vi "soundwave_generator_v06_complete_user.vi"() -> ()   [LabVIEW 2019]
uses:
  global.vi
panel:
  in  "Choice Equal":bool
  in  "Choice 2":bool
  in  "Choice 1":bool
  out "choice 2 LED":bool
  out "choice 1 LED":bool
  in  "Repeat Trial":bool
  out "Trial":i32
  out "Protocol Progression":i32(slide) scale=0.0..90.0
  out "Red Light":bool
  out "Green Light":bool
  out "Sound number":string
  # "Trial #"
  # "Which sound did you prefer?"
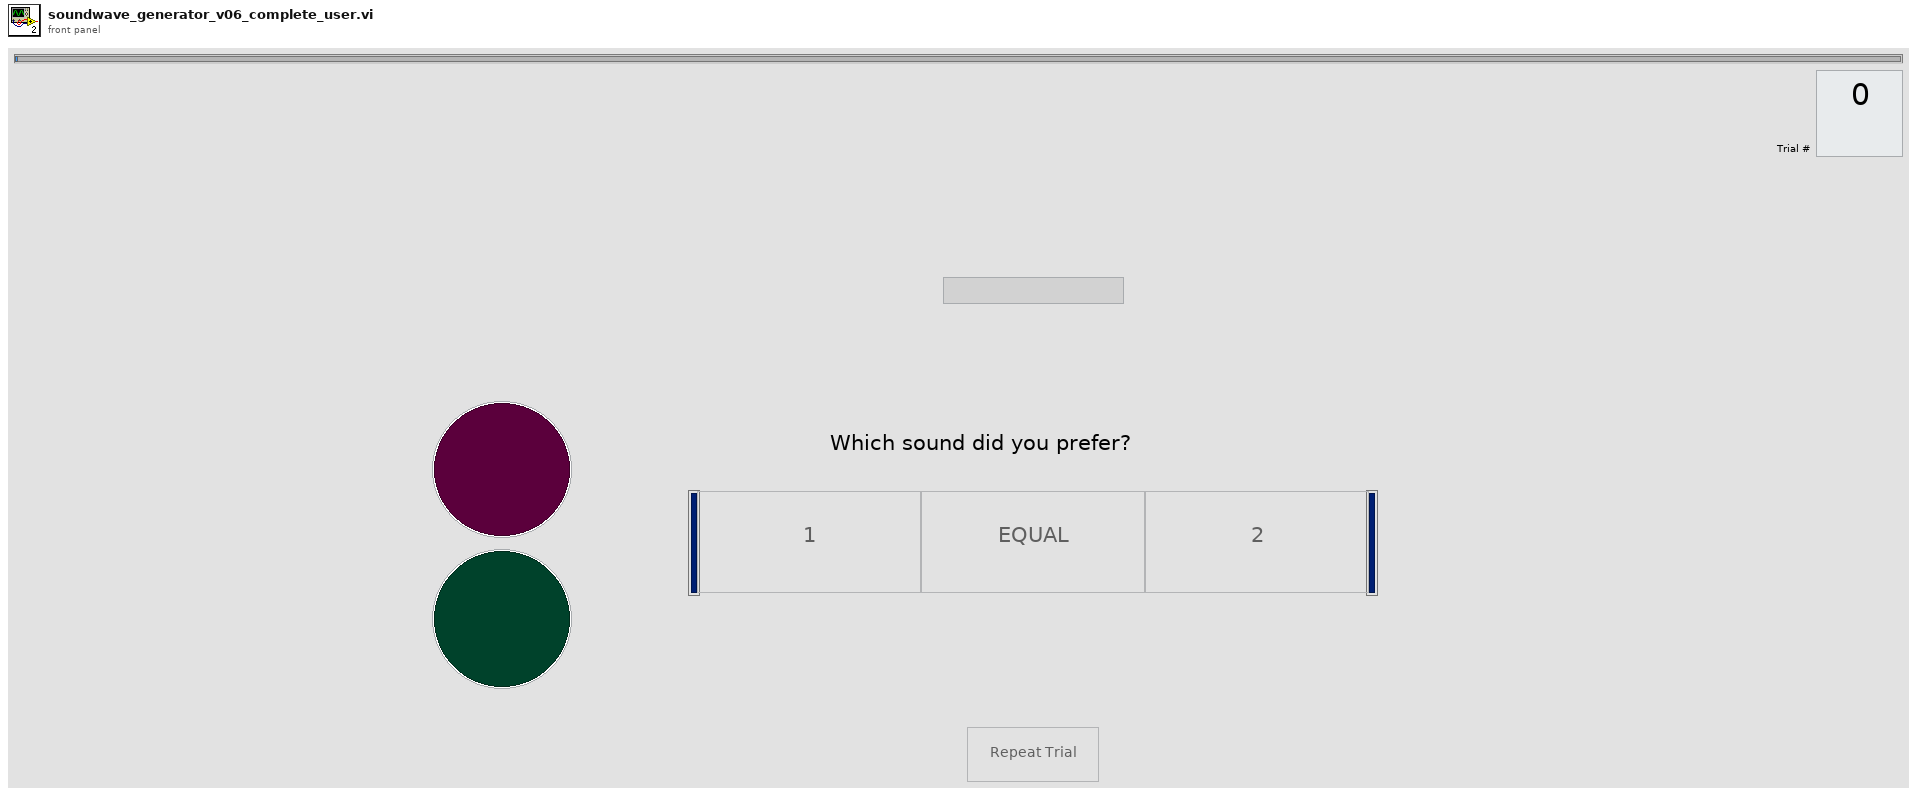
[diagram p1: front panel]
types:
  T1 = enum8{"Enabled", "Disabled", "Disabled and Grayed Out"}
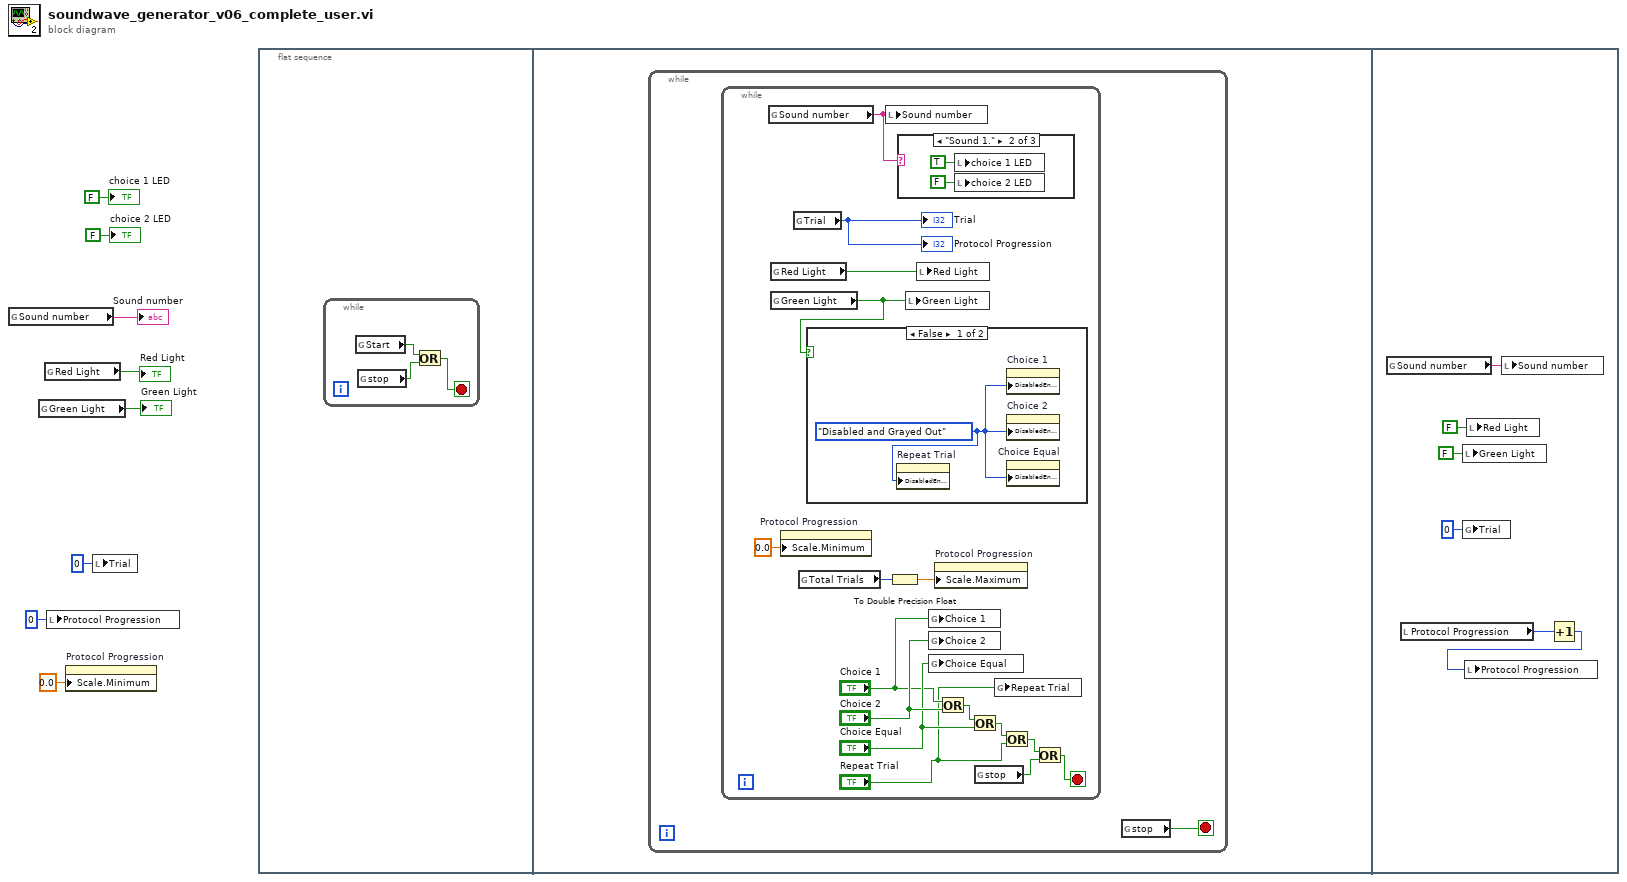
[diagram p0: block diagram]
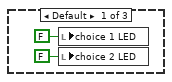
[diagram p2: hidden frame]
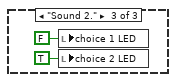
[diagram p3: hidden frame]
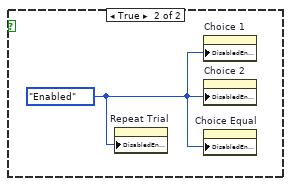
[diagram p4: hidden frame]
diagram:
  n1 = global read "global.vi" "Sound number"() -> (→"Sound number":string)
  n2 = global read "global.vi" "Green Light"() -> (→"Green Light":bool)
  n3 = global read "global.vi" "Red Light"() -> (→"Red Light":bool)
  n4 = local write "Protocol Progression"(0 ("Protocol Progression")) -> ()
  n5 = property on="Protocol Progression" class="Slide (strict)"("Scale.Minimum"=0.0 ("Scale.Range:Minimum")) -> ()  [unwired: 2 in, 2 out]
  n6 = local write "Trial"(0 ("Trial")) -> ()
  n7 = flat-sequence {
    frame #0 {
      n8 = while {
        stop <- w11 stop-if-true
        n9 = global read "global.vi" "Start"() -> (w9:bool)
        n10 = global read "global.vi" "stop"() -> (w10:bool)
        n11 = Or(x=w9, y=w10) -> (x .or. y?=w11:bool)
      }
    }
    frame #1 {
      n12 = while {
        stop <- w12 stop-if-true
        n13 = while {
          stop <- w28 stop-if-true
          n14 = global read "global.vi" "Sound number"() -> (w14:string)
          n15 = global read "global.vi" "Red Light"() -> (w23:bool)
          n16 = global read "global.vi" "Green Light"() -> (w13:bool)
          n17 = property on="Protocol Progression" class="Slide (strict)"("Scale.Minimum"=0.0 ("Scale.Range:Minimum")) -> ()  [unwired: 2 in, 2 out]
          n18 = global read "global.vi" "Trial"() -> (→"Protocol Progression" →"Trial":i32)
          n19 = global read "global.vi" "Total Trials"() -> (w22:i32)
          n20 = case shown="False" w13 {
            frame False {
              w35 = T1."Disabled and Grayed Out" ("Disabled")
              n21 = property on="Repeat Trial" class="Bool"("DisabledEnum"=w35) -> ()  [unwired: 2 in, 2 out]
              n22 = property on="Choice 1" class="Bool"("DisabledEnum"=w35) -> ()  [unwired: 2 in, 2 out]
              n23 = property on="Choice 2" class="Bool"("DisabledEnum"=w35) -> ()  [unwired: 2 in, 2 out]
              n24 = property on="Choice Equal" class="Bool"("DisabledEnum"=w35) -> ()  [unwired: 2 in, 2 out]
            }
            frame True {
              w36 = T1."Enabled" ("Disabled")
              n25 = property on="Repeat Trial" class="Bool"("DisabledEnum"=w36) -> ()  [unwired: 2 in, 2 out]
              n26 = property on="Choice 1" class="Bool"("DisabledEnum"=w36) -> ()  [unwired: 2 in, 2 out]
              n27 = property on="Choice 2" class="Bool"("DisabledEnum"=w36) -> ()  [unwired: 2 in, 2 out]
              n28 = property on="Choice Equal" class="Bool"("DisabledEnum"=w36) -> ()  [unwired: 2 in, 2 out]
            }
          }
          n29 = local write "Sound number"(w14) -> ()
          n30 = To Double Precision Float(number=w22) -> (double precision float=w21:dbl)
          n31 = case shown="\"Sound 1.\"" w14 {
            frame Default {
              n32 = local write "choice 1 LED"(FALSE ("choice 1 LED")) -> ()
              n33 = local write "choice 2 LED"(FALSE ("choice 2 LED")) -> ()
            }
            frame "Sound 1." {
              n34 = local write "choice 1 LED"(TRUE ("choice 1 LED")) -> ()
              n35 = local write "choice 2 LED"(FALSE ("choice 2 LED")) -> ()
            }
            frame "Sound 2." {
              n36 = local write "choice 1 LED"(FALSE ("choice 1 LED")) -> ()
              n37 = local write "choice 2 LED"(TRUE ("choice 2 LED")) -> ()
            }
          }
          n38 = local write "Green Light"(w13) -> ()
          n39 = local write "Red Light"(w23) -> ()
          n40 = global write "global.vi" "Choice 1"("Choice 1") -> ()
          n41 = global write "global.vi" "Choice 2"("Choice 2") -> ()
          n42 = global write "global.vi" "Choice Equal"("Choice Equal") -> ()
          n43 = property on="Protocol Progression" class="Slide (strict)"("Scale.Maximum"=w21) -> ()  [unwired: 2 in, 2 out]
          n44 = Or(x="Choice 1", y="Choice 2") -> (x .or. y?=w27:bool)
          n45 = Or(x=w27, y="Choice Equal") -> (x .or. y?=w18:bool)
          n46 = global read "global.vi" "stop"() -> (w26:bool)
          n47 = global write "global.vi" "Repeat Trial"("Repeat Trial") -> ()
          n48 = Or(x=w18, y="Repeat Trial") -> (x .or. y?=w17:bool)
          n49 = Or(x=w17, y=w26) -> (x .or. y?=w28:bool)
        }
        n50 = global read "global.vi" "stop"() -> (w12:bool)
      }
    }
    frame #2 {
      n51 = global read "global.vi" "Sound number"() -> (w42:string)
      n52 = local read "Protocol Progression"() -> (w38:i32)
      n53 = local write "Green Light"(FALSE ("Green Light")) -> ()
      n54 = global write "global.vi" "Trial"(0 ("Trial")) -> ()
      n55 = local write "Red Light"(FALSE ("Red Light")) -> ()
      n56 = local write "Sound number"(w42) -> ()
      n57 = Increment(x=w38) -> (x+1=w37:i32)
      n58 = local write "Protocol Progression"(w37) -> ()
    }
  }
  "choice 1 LED" <- FALSE ("choice 1 LED")
  "choice 2 LED" <- FALSE ("choice 2 LED")
